vi "PERTRAS Editor.vi"() -> ()   [LabVIEW 2010]
panel:
  out "Achtung":string
  in  "Zykluslängen":bool
  in  "mod2":bool
  in  "mod1":bool
  in  "mod0":bool
  in  "neue Methode":bool
  in  "Änderungen speichern":bool
  in  "Stopp":bool
  in  "Methode laden":bool
  in  "Methode schließen":bool
  out "new picture":picture
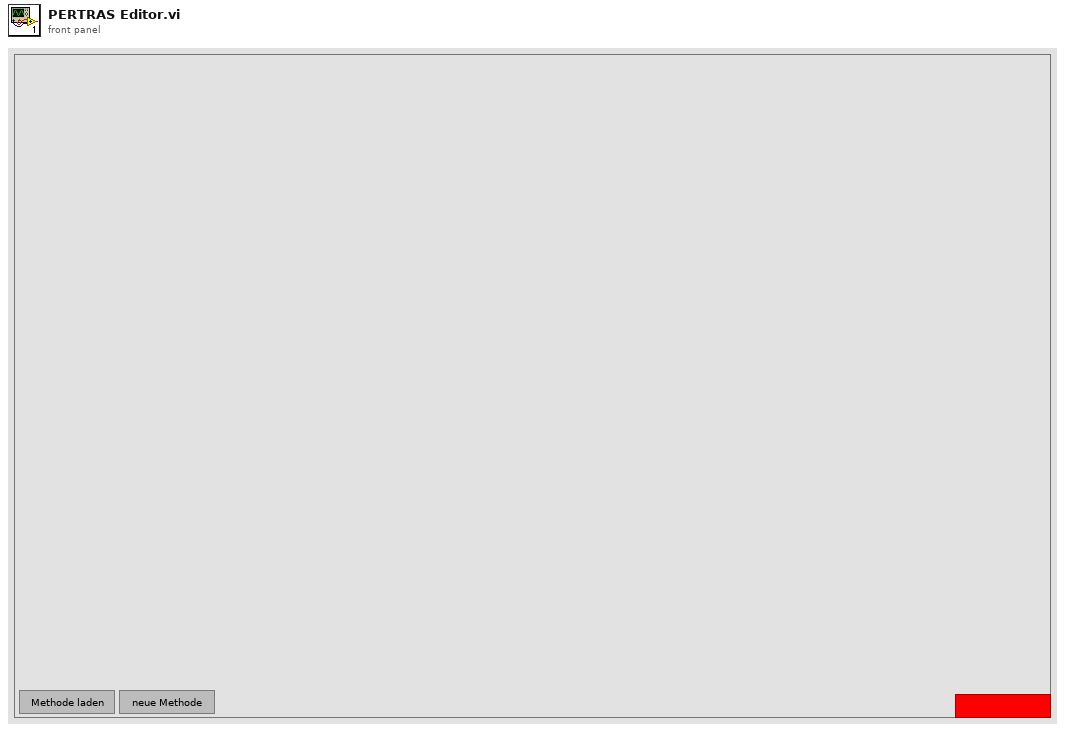
[diagram p1: front panel]
types:
  T1 = enum16{"open", "replace", "create", "open or create", "replace or create", "replace or create with confirmation"}
  T2 = typedef "imagedata.ctl" = cluster{"image type":i32, "image depth":i32, "image":u8[], "mask":u8[], "colors":u32[], "Rectangle":cluster{"left":i16, "top":i16, "right":i16, "bottom":i16}}
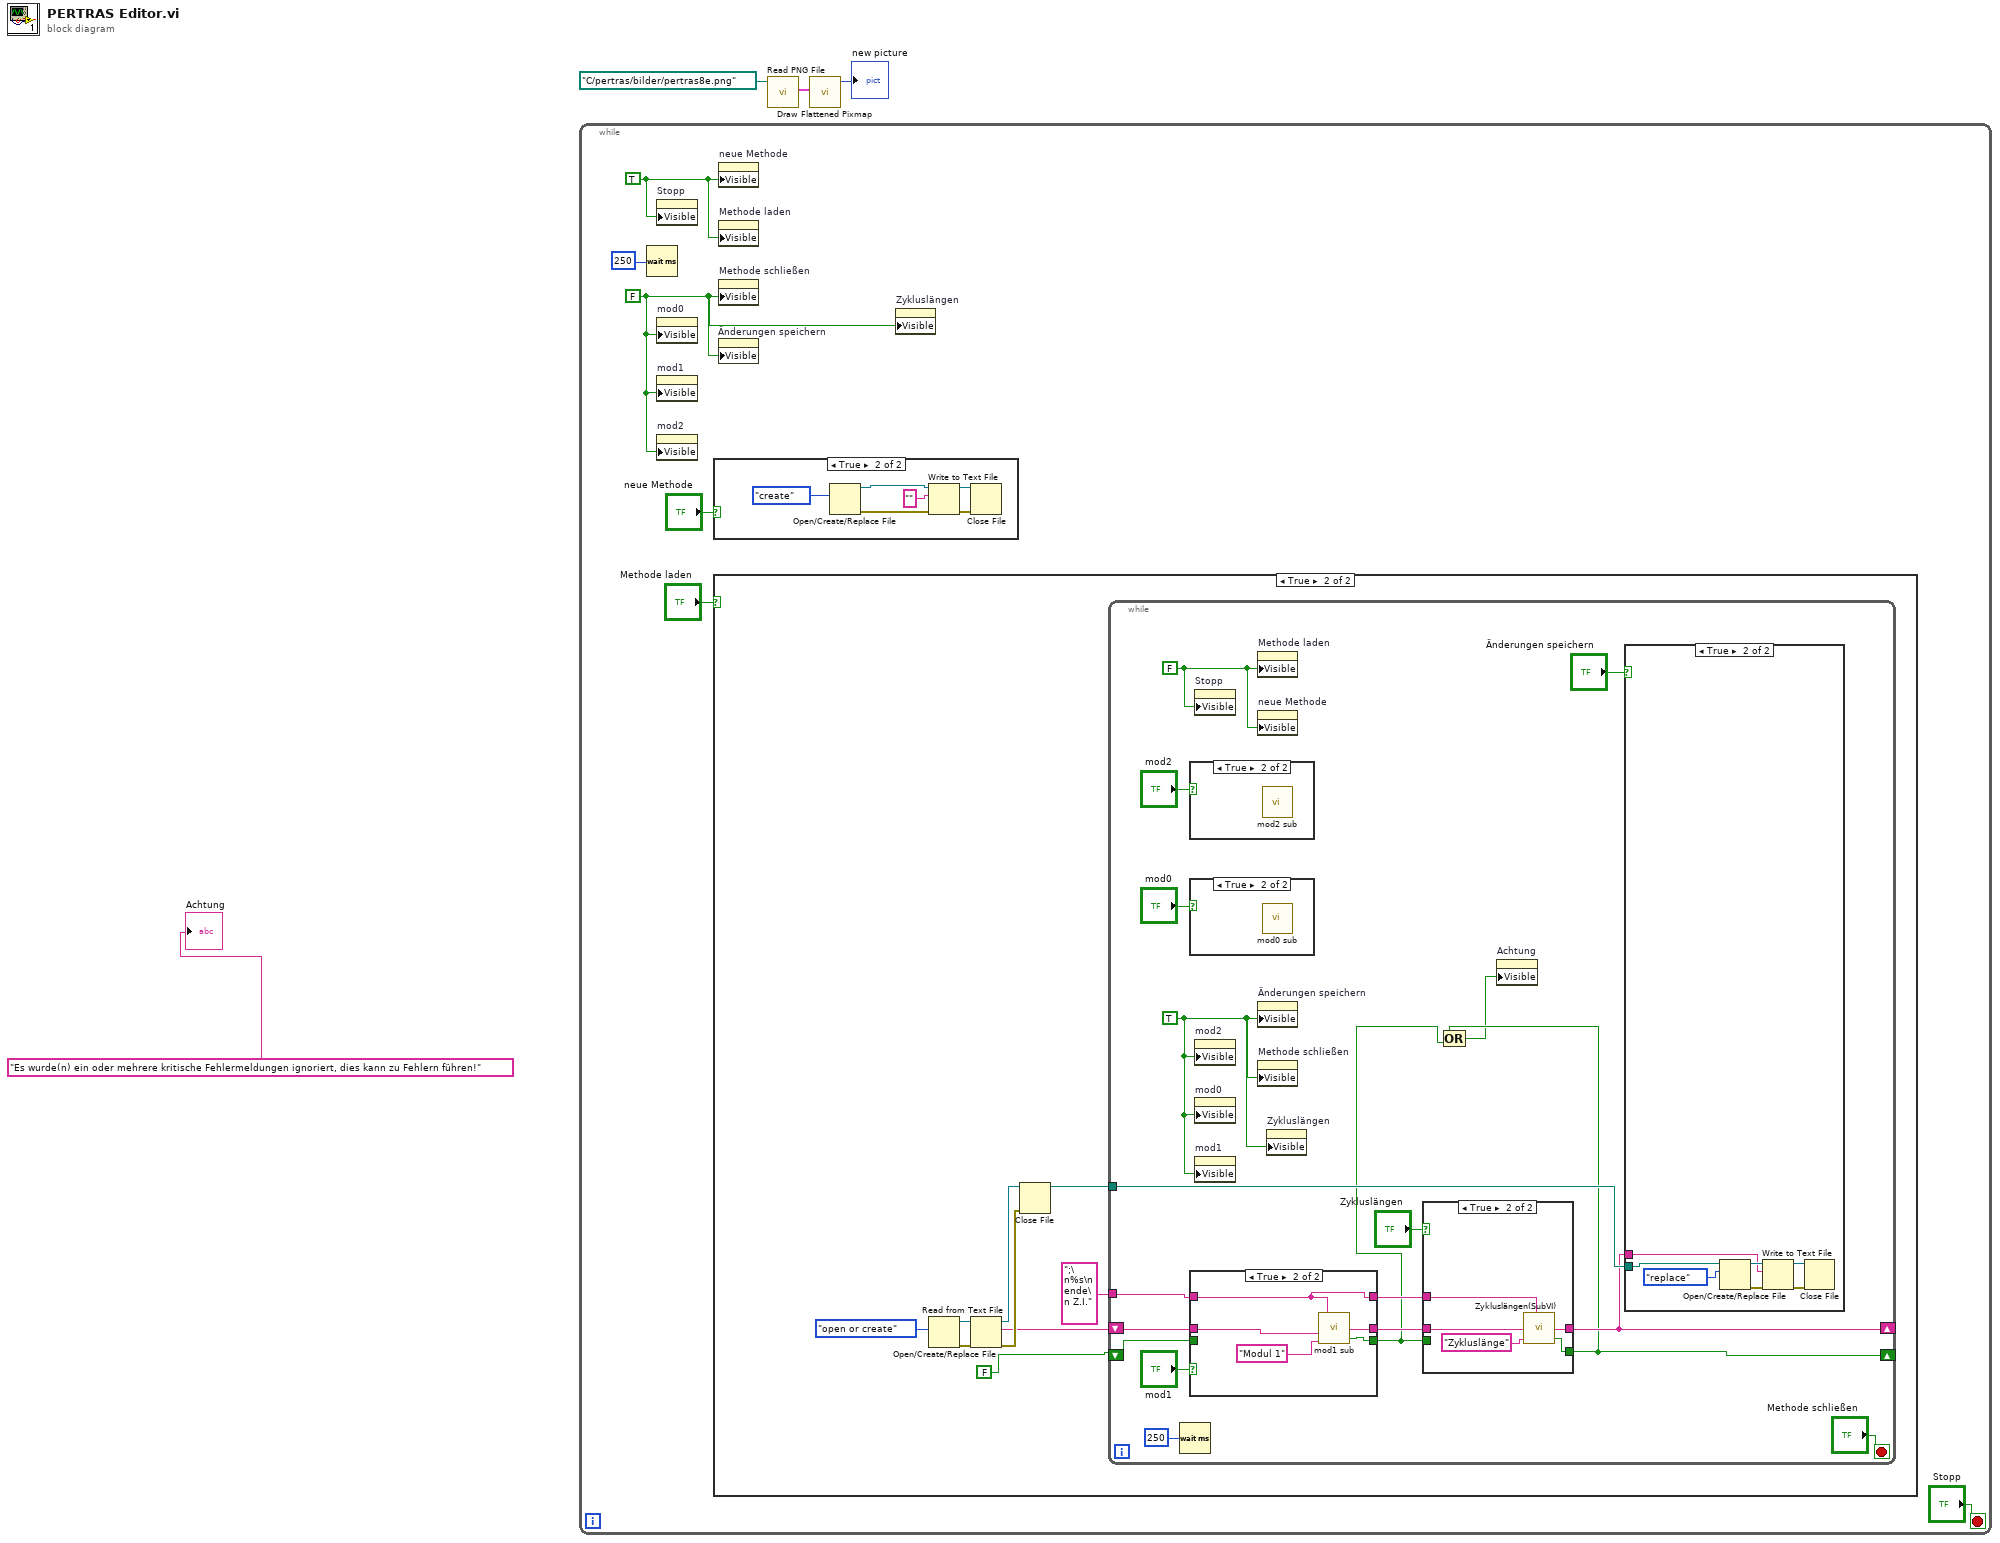
[diagram p0: block diagram]
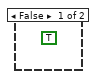
[diagram p2: hidden frame]
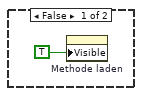
[diagram p3: hidden frame]
diagram:
  n1 = while {
    stop <- "Stopp" stop-if-true
    w8 = TRUE
    w5 = FALSE ("Sichtbar")
    n2 = Wait (ms)(milliseconds to wait=u32 250 ("Zu wartende ms")) -> ()  [unwired: 1 out]
    n3 = property on="Stopp" class="Bool."("Visible"=w8) -> ()  [unwired: 2 in, 2 out]
    n4 = property on="mod0" class="Bool."("Visible"=w5) -> ()  [unwired: 2 in, 2 out]
    n5 = property on="mod1" class="Bool."("Visible"=w5) -> ()  [unwired: 2 in, 2 out]
    n6 = property on="mod2" class="Bool."("Visible"=w5) -> ()  [unwired: 2 in, 2 out]
    n7 = case shown="True" "neue Methode" {
      frame False {
        (unwired) TRUE
      }
      frame True {
        n8 = Open/Create/Replace File(operation (0:open)=T1."create" ("Operation (0:Öffnen)")) -> (refnum out=w14:refnum<file>, error out=w13:errorcluster)  [unwired: 5 in, 1 out]
        n9 = Write to Text File(file (use dialog)=w14, text="" ("Text"), error in=w13) -> (refnum out=w15:refnum<file>, error out=w16:errorcluster)  [unwired: 1 in, 1 out]
        n10 = Close File(refnum=w15, error in=w16) -> ()  [unwired: 2 out]
      }
    }
    n11 = case shown="True" "Methode laden" {
      frame False {
        n12 = property on="Methode laden" class="Bool."("Visible"=TRUE ("Sichtbar")) -> ()  [unwired: 2 in, 2 out]
      }
      frame True {
        n13 = Open/Create/Replace File(operation (0:open)=T1."open or create" ("Operation (0:Öffnen)")) -> (refnum out=w26:refnum<file>, error out=w25:errorcluster)  [unwired: 5 in, 1 out]
        n14 = Read from Text File(file (use dialog)=w26, error in=w25) -> (refnum out=w24:refnum<file>, text=w21:string, error out=w23:errorcluster)  [unwired: 2 in, 1 out]
        n15 = Close File(refnum=w24, error in=w23) -> (path=w22:path)  [unwired: 1 out]
        n16 = while {
          tunnel: w22 -> [w43]
          tunnel: ";\n%s\n ende\n Z.I." ("Trennzeichen") -> [w36]
          shift-right: [w35] -> _
          shift-left: w21 -> [w37]
          shift-right: [w30] -> _
          shift-left: FALSE ("Sperre") -> [w28]
          stop <- "Methode schließen" stop-if-true
          w27 = TRUE ("Sichtbar")
          w42 = FALSE ("Sichtbar")
          n17 = Wait (ms)(milliseconds to wait=u32 250 ("Zu wartende ms")) -> ()  [unwired: 1 out]
          n18 = case shown="True" "mod2" {
            frame False {
            }
            frame True {
              n19 = call "mod2 sub.vi"() -> ()  [unwired: 1 in, 1 out]
            }
          }
          n20 = case shown="True" "mod0" {
            frame False {
            }
            frame True {
              n21 = call "mod0 sub.vi"() -> ()  [unwired: 1 in, 2 out]
            }
          }
          n22 = case shown="True" "mod1" {
            tunnel: w37 -> [w55 w60]
            tunnel: w36 -> [w54 w57]
            tunnel: [w55 w59] -> w34
            tunnel: [w54 w57] -> w33
            tunnel: w28 -> [w53 _]
            tunnel: [w53 w56] -> w31
            frame False {
            }
            frame True {
              n23 = call "mod1 sub.vi"("Modulname"="Modul 1", "Daten"=w60, "Format"=w57) -> ("Sperre"=w56:bool, "Ausgang"=w59:string)  [unwired: 2 in]
            }
          }
          n24 = property on="Stopp" class="Bool."("Visible"=w42) -> ()  [unwired: 2 in, 2 out]
          n25 = property on="mod2" class="Bool."("Visible"=w27) -> ()  [unwired: 2 in, 2 out]
          n26 = property on="mod0" class="Bool."("Visible"=w27) -> ()  [unwired: 2 in, 2 out]
          n27 = property on="mod1" class="Bool."("Visible"=w27) -> ()  [unwired: 2 in, 2 out]
          n28 = property on="Methode laden" class="Bool."("Visible"=w42) -> ()  [unwired: 2 in, 2 out]
          n29 = property on="neue Methode" class="Bool."("Visible"=w42) -> ()  [unwired: 2 in, 2 out]
          n30 = property on="Änderungen speichern" class="Bool."("Visible"=w27) -> ()  [unwired: 2 in, 2 out]
          n31 = property on="Methode schließen" class="Bool."("Visible"=w27) -> ()  [unwired: 2 in, 2 out]
          n32 = property on="Zykluslängen" class="Bool."("Visible"=w27) -> ()  [unwired: 2 in, 2 out]
          n33 = case shown="True" "Zykluslängen" {
            tunnel: [w47 w51] -> w35
            tunnel: w34 -> [w47 w52]
            tunnel: w33 -> [_ w50]
            tunnel: w31 -> [w46 _]
            tunnel: [w46 w48] -> w30
            frame False {
            }
            frame True {
              n34 = call "Zykluslängen(SubVI).vi"("Formatierung"=w50, "Daten"=w52, "Modulname"="Zykluslänge") -> ("Ausgang"=w51:string, "Sperre"=w48:bool)  [unwired: 3 in]
            }
          }
          n35 = Compound Arithmetic op=OR(w30, w31) -> (w29:bool)
          n36 = property on="Achtung" class="Str"("Visible"=w29) -> ()  [unwired: 2 in, 2 out]
          n37 = case shown="True" "Änderungen speichern" {
            tunnel: w43 -> [_ w62]
            tunnel: w35 -> [_ w61]
            frame False {
            }
            frame True {
              n38 = Open/Create/Replace File(file path (use dialog)=w62, operation (0:open)=T1."replace" ("Operation (0:Öffnen)")) -> (refnum out=w66:refnum<file>, error out=w64:errorcluster)  [unwired: 4 in, 1 out]
              n39 = Write to Text File(file (use dialog)=w66, text=w61, error in=w64) -> (refnum out=w67:refnum<file>, error out=w63:errorcluster)  [unwired: 1 in, 1 out]
              n40 = Close File(refnum=w67, error in=w63) -> ()  [unwired: 2 out]
            }
          }
        }
      }
    }
    n41 = property on="neue Methode" class="Bool."("Visible"=w8) -> ()  [unwired: 2 in, 2 out]
    n42 = property on="Methode laden" class="Bool."("Visible"=w8) -> ()  [unwired: 2 in, 2 out]
    n43 = property on="Methode schließen" class="Bool."("Visible"=w5) -> ()  [unwired: 2 in, 2 out]
    n44 = property on="Änderungen speichern" class="Bool."("Visible"=w5) -> ()  [unwired: 2 in, 2 out]
    n45 = property on="Zykluslängen" class="Bool."("Visible"=w5) -> ()  [unwired: 2 in, 2 out]
  }
  n46 = call <vilib>:"Read PNG File.vi"("path to PNG file"=path "C:/pertras/bilder/pertras8e.png") -> ("image data"=w2:T2)  [unwired: 8 in, 2 out]
  n47 = call <vilib>:"Draw Flattened Pixmap.vi"("image data"=w2) -> ("new picture"=→"new picture":picture)  [unwired: 8 in]
  "Achtung" <- "Es wurde(n) ein oder mehrere kritische Fehlermeldungen ignoriert, dies kann zu Fehlern führen!"
